vi "Register For Test Cases Found Event.vi"(8 "error in (no error)":errorcluster, 11 "Test Finder In":refnum<class "Test Finder.lvclass">) -> (0 "error out":errorcluster, 2 "Test Cases Found Registration":refnum<event-registration>, 3 "Test Finder Out":refnum<class "Test Finder.lvclass">)   [LabVIEW 2020, in "Test Finder.lvclass"]
uses:
  Test Finder.lvclass
  Test Finder.lvclass/Test Finder.ctl
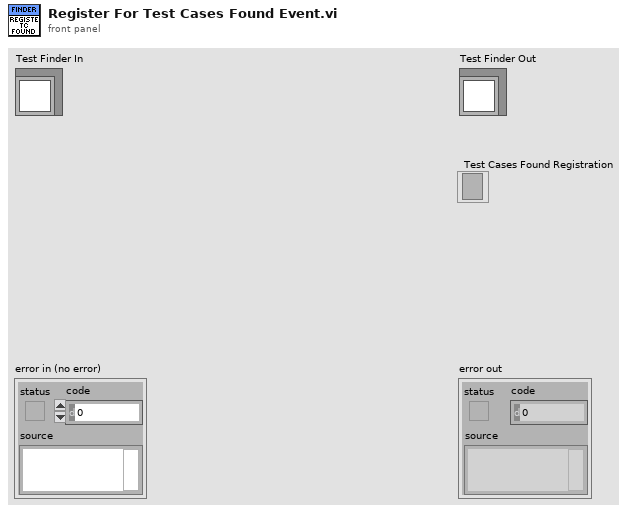
[diagram p1: front panel]
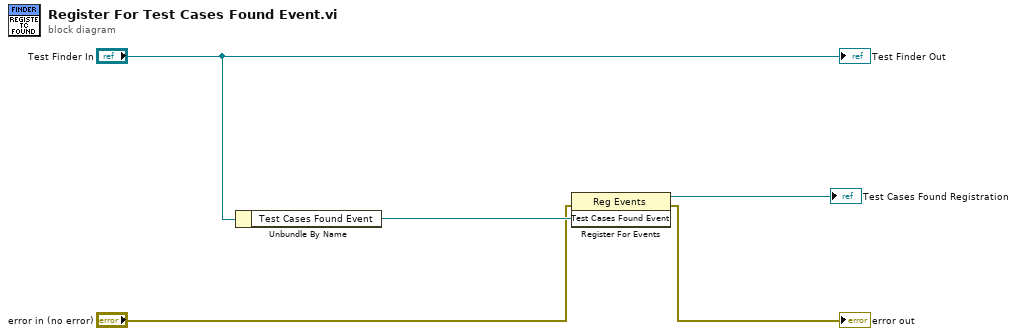
[diagram p0: block diagram]
diagram:
  n1 = Unbundle By Name("Test Finder In") -> ("Test Cases Found Event"=w4:refnum<user-event>)
  n2 = register-events(error in="error in (no error)", w4) -> (reference out=→"Test Cases Found Registration":refnum<event-registration>, error out=→"error out":errorcluster)  [unwired: 1 in]
  "Test Finder Out" <- "Test Finder In"
